vi "Update Image Control.vi"(8 "error in (no error)":errorcluster, 10 "Image Indicator":refnum<vi>, 11 "ImageHandler in":refnum<class "ImageHandler.lvclass">) -> (0 "error out":errorcluster, 3 "ImageHandler out":refnum<class "ImageHandler.lvclass">)   [LabVIEW 2022 SP3, in "ImageHandler.lvlib" / "ImageHandler.lvclass"]
uses:
  ImageHandler.lvclass
  ImageHandler.lvclass/ImageHandler.ctl
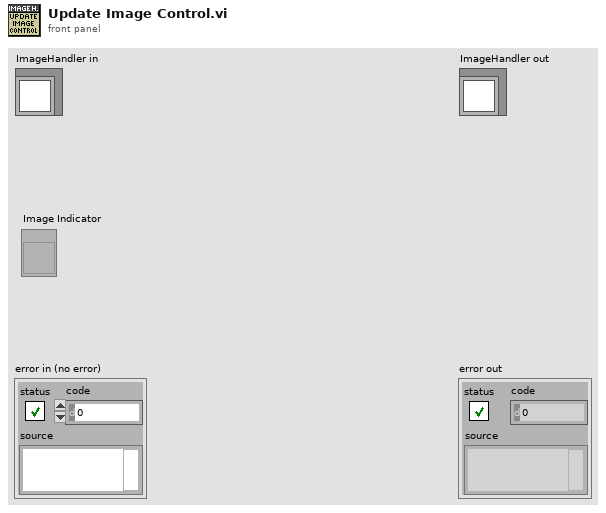
[diagram p1: front panel]
types:
  T1 = typedef "IMAQ Image.ctl" = refnum<image>
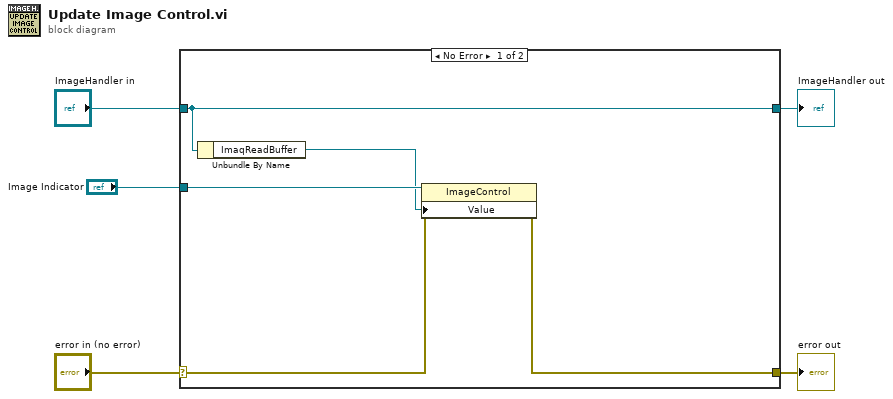
[diagram p0: block diagram]
diagram:
  n1 = case shown="No Error" "error in (no error)" {
    selector: "error in (no error)" -> [w10 w12]
    tunnel: [w8 w12] -> w4
    tunnel: [w9 w11] -> w2
    tunnel: "ImageHandler in" -> [w9 w11]
    tunnel: "Image Indicator" -> [w7 _]
    frame No Error {
      n2 = Unbundle By Name(w9) -> ("ImaqReadBuffer"=w6:T1)
      n3 = property class="ImageControl"(reference=w7, error in=w10, "Value"=w6) -> (error out=w8:errorcluster)  [unwired: 1 out]
    }
    frame Error {
    }
  }
  "error out" <- w4
  "ImageHandler out" <- w2
